vi "Tektronix MSO5X Series Read Horizontal Settings.vi"() -> ()   [LabVIEW 2021]
doc: "This example VI illustrates how to configure and query horizontal properties."
uses:
  <instrlib>/Tektronix MSO5X Series/Tektronix MSO5X Series.lvlib
panel:
  in  "error in":errorcluster
  out "error out":errorcluster
  in  "Maximum Record Length":dbl=250000000.0 format="%#_6e"
  in  "Sample Rate":dbl=3125000000.0
  in  "Control Type":i32(ring) items=["Horizontal Scale", "Record Length"]
  out "Division Number":i32
  out "Timebase Duration (s)":dbl
  out "Interpolation Ratio":dbl
  in  "Tektronix Scope":refnum<visa-resource-name>
  # "(c) 2023  National Instruments Corporation.  ALL RIGHTS RESERVED."
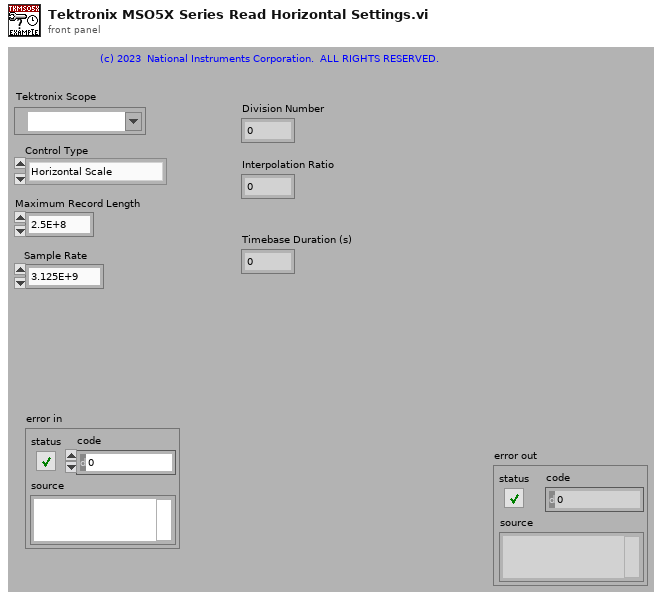
[diagram p1: front panel]
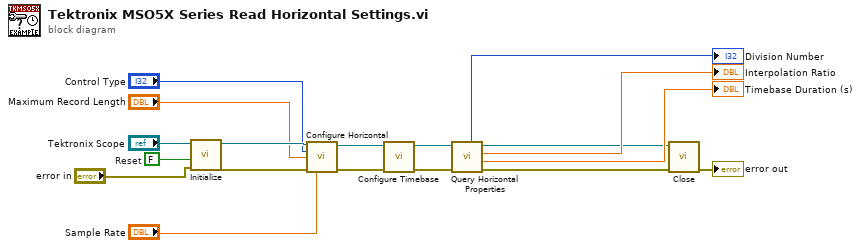
[diagram p0: block diagram]
diagram:
  w17 = FALSE  # Reset
  n1 = call <instrlib>:"Initialize.vi"("error in (no error)"="error in", "Reset (True)"=w17, "VISA resource name"="Tektronix Scope") -> ("error out"=w15:errorcluster, "VISA resource name out"=w16:refnum<visa-resource-name>)  [unwired: 7 in]
  n2 = call <instrlib>:"Configure Horizontal.vi"("VISA resource name"=w16, "Control Type (0: Horizontal Scale)"="Control Type", "Maximum Record Length (2.5E+8)"="Maximum Record Length", "error in (no error)"=w15, "Sample Rate (3.125E+9)"="Sample Rate") -> ("VISA resource name out"=w6:refnum<visa-resource-name>, "error out"=w5:errorcluster)  [unwired: 9 in]
  n3 = call <instrlib>:"Configure Timebase.vi"("error in (no error)"=w5, "VISA resource name"=w6) -> ("error out"=w4:errorcluster, "VISA resource name out"=w3:refnum<visa-resource-name>)  [unwired: 8 in]
  n4 = call <instrlib>:"Query Horizontal Properties.vi"("error in (no error)"=w4, "VISA resource name"=w3) -> ("error out"=w7:errorcluster, "Timebase Duration (s)"=→"Timebase Duration (s)":dbl, "Interpolation Ratio"=→"Interpolation Ratio":dbl, "VISA resource name out"=w8:refnum<visa-resource-name>, "Division Number"=→"Division Number":i32)  [unwired: 5 in]
  n5 = call <instrlib>:"Close.vi"("error in (no error)"=w7, "VISA resource name"=w8) -> ("error out"=→"error out":errorcluster)  [unwired: 9 in]
